vi "Set 3D Properties.vi"(8 "error in (no error)":errorcluster, 10 "3D":T1={"Enable 3D"=FALSE, "LightStyle"=enum."Realistic", "PointGapDepth"=150, "PointDepth"=120, "Perspective"=6, "WallWidth"=0}, 11 ".NET MSChart ChartArea":refnum<k24>) -> (0 "error out":errorcluster, 3 ".NET MSChart ChartArea":refnum<k24>)   [LabVIEW 2015, in "Graph Extensions MSChart.lvlib"]
uses:
  Graph Extensions MSChart.lvlib
  System.Windows.Forms.DataVisualization
  Controls/3D.ctl
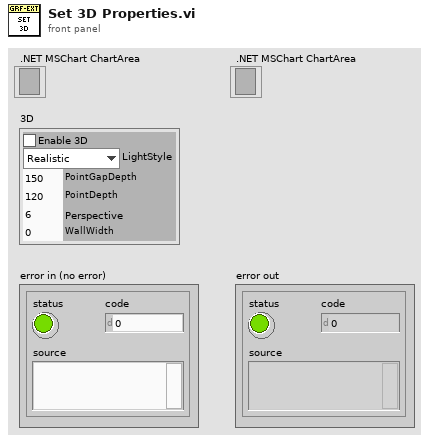
[diagram p1: front panel]
types:
  T1 = typedef "Graph Extensions MSChart.lvlib/3D.ctl" = cluster{"Enable 3D":bool, "LightStyle":enum16{"None", "Simplistic", "Realistic"}, "PointGapDepth":i32, "PointDepth":i32, "Perspective":i32, "WallWidth":i32}
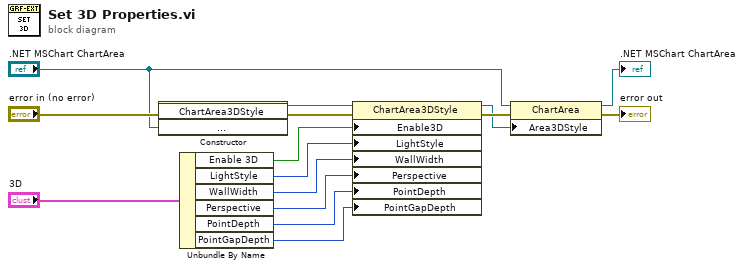
[diagram p0: block diagram]
diagram:
  n1 = constructor class="ChartArea3DStyle"(error in="error in (no error)", "chartArea"=".NET MSChart ChartArea") -> (reference out=w15:refnum<k24>, error out=w6:errorcluster)  [unwired: 2 in, 2 out]
  n2 = Unbundle By Name("3D") -> ("Enable 3D"=w13:bool, "LightStyle"=w12:enum16{"None", "Simplistic", "Realistic"}, "WallWidth"=w11:i32, "Perspective"=w10:i32, "PointDepth"=w9:i32, "PointGapDepth"=w8:i32)
  n3 = property class="ChartArea3DStyle"(reference=w15, error in=w6, "Enable3D"=w13, "LightStyle"=w12, "WallWidth"=w11, "Perspective"=w10, "PointDepth"=w9, "PointGapDepth"=w8) -> (reference out=w3:refnum<k24>, error out=w4:errorcluster)
  n4 = property class="ChartArea"(reference=".NET MSChart ChartArea", error in=w4, "Area3DStyle"=w3) -> (reference out=→".NET MSChart ChartArea":refnum<k24>, error out=→"error out":errorcluster)
